vi "REQ Config Measurement.vi"(8 "error in":errorcluster, 10 "Meas Setting":T1={"Function (0: DC Voltage)"=0, "Manual Resolution (5.5 Digits)"=5.5, "Manual Range (1.00)"=1.0, "Enable Auto Range (T: Enable)"=TRUE} {"Manual Range (1.00)" format="%_3f"; "Manual Resolution (5.5 Digits)" items=["4.5"=4.5, "5.5"=5.5, "6.5"=6.5]; "Function (0: DC Voltage)" items=["DC Voltage", "AC Voltage", "2 - Wire Resistance", "4 - Wire Resistance", "DC Current", "AC Current", "Frequency", "Period", "Continuity", "Diode Checking", "VDC:VDC Ratio", "Temperature", "Capacitance"]}) -> (0 "error out":errorcluster)   [LabVIEW 2021, in "DMM.lvlib"]
doc: "_____\nCreated using DQMH Event Scripter 6.1.0.128."
uses:
  DMM.lvlib
  REQ Config Measurement Argument--cluster.ctl
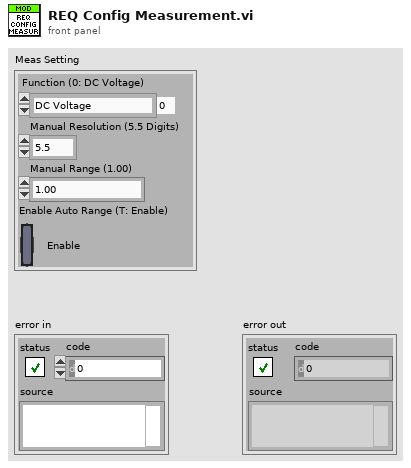
[diagram p1: front panel]
types:
  T1 = cluster{"Function (0: DC Voltage)":u16, "Manual Resolution (5.5 Digits)":dbl, "Manual Range (1.00)":dbl, "Enable Auto Range (T: Enable)":bool}
  T2 = typedef "DMM.lvlib/REQ Config Measurement Argument--cluster.ctl" = cluster{"Meas Setting":cluster{"Function (0: DC Voltage)":u16, "Manual Resolution (5.5 Digits)":dbl, "Manual Range (1.00)":dbl, "Enable Auto Range (T: Enable)":bool}}
  T3 = typedef "DMM.lvlib/Request Events--cluster.ctl" = cluster{"Stop Module":refnum<user-event>, "Show Panel":refnum<user-event>, "Hide Panel":refnum<user-event>, "Get Module Execution Status":refnum<user-event>, "Show Diagram":refnum<user-event>, "REQ Initialize Hardware":refnum<user-event>, "REQ Close Ref":refnum<user-event>, "REQ Config Measurement":refnum<user-event>, "REQ Read Single Meas":refnum<user-event>, "REQ Self Test":refnum<user-event>, "REQ Retry DMM":refnum<user-event>}
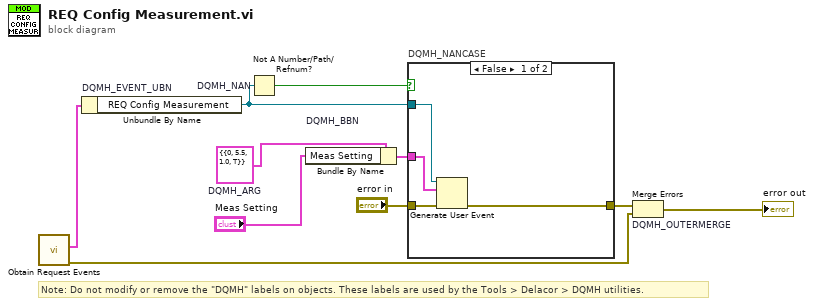
[diagram p0: block diagram]
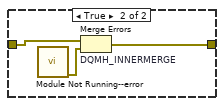
[diagram p2: hidden frame]
diagram:
  w4 = T2 {"Meas Setting"={"Function (0: DC Voltage)"=0, "Manual Resolution (5.5 Digits)"=5.5, "Manual Range (1.00)"=1.0, "Enable Auto Range (T: Enable)"=TRUE}}  # DQMH_ARG
  # "Note: Do not modify or remove the \"DQMH\" labels on objects. These labels are used by the Tools > Delacor > DQMH utilities."
  n1 = call "Obtain Request Events.vi"() -> ("error out"=w2:errorcluster, "DMM Request Events"=w1:T3)  [unwired: 10 in]
  n2 = Unbundle By Name "DQMH_EVENT_UBN"(w1) -> ("REQ Config Measurement"=w6:refnum<user-event>)
  n3 = Not A Number/Path/Refnum? "DQMH_NAN"(number/path/refnum=w6) -> (NaN/Path/Refnum?=w7:bool)
  n4 = Bundle By Name "DQMH_BBN"(cluster=w4, "Meas Setting"="Meas Setting") -> (w8:T2)
  n5 = case "DQMH_NANCASE" shown="False" w7 {
    tunnel: "error in" -> [w14 w17]
    tunnel: [w13 w16] -> w5
    tunnel: w6 -> [w12 _]
    tunnel: w8 -> [w11 _]
    frame False {
      n6 = Generate User Event(user event=w12, event data cluster=w11, error in=w14) -> (error out=w13:errorcluster)  [unwired: 1 in, 1 out]
    }
    frame True {
      n7 = call "Module Not Running--error.vi"() -> ("error out"=w15:errorcluster)  [unwired: 11 in]
      n8 = Merge Errors "DQMH_INNERMERGE"(w17, w15) -> (w16:errorcluster)
    }
  }
  n9 = Merge Errors "DQMH_OUTERMERGE"(w5, w2) -> (→"error out":errorcluster)
